vi "RangeDisplay.vi"(7 "Unit":T2, 9 "Range":T1, 11 "error in (no error)":errorcluster) -> (6 "Display":string, 10 "Range":T1, 15 "error out":errorcluster)   [LabVIEW 2014, in "FH 55.lvlib"]
doc: "Dieses VI gibt für die Range (abhängig von der Einheit) denn Zahlenwert für den Display zurück.\n\n\nThis VI gives for the range (depending on the unit) a numerical value for the display back."
uses:
  FH 55.lvlib
  TypeDef/Range.ctl
  TypeDef/Unit.ctl
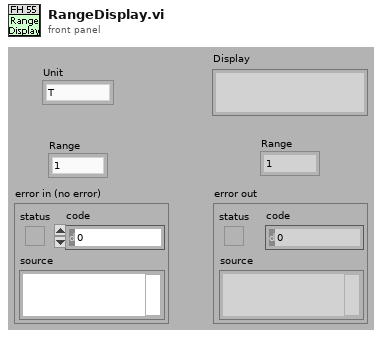
[diagram p1: front panel]
types:
  T1 = typedef "FH 55.lvlib/Range.ctl" = enum16{"1", "2", "3", "4", "5", "6", "7"}
  T2 = typedef "FH 55.lvlib/Unit.ctl" = enum16{"T", "G", "A/m"}
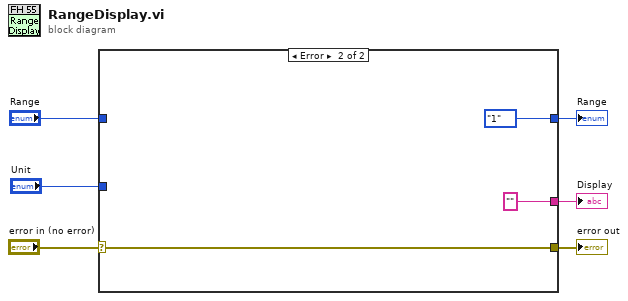
[diagram p0: block diagram]
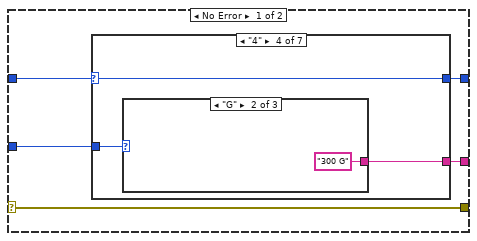
[diagram p2: hidden frame]
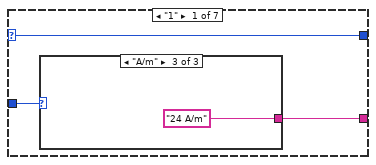
[diagram p3: hidden frame]
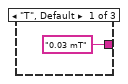
[diagram p4: hidden frame]
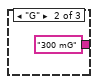
[diagram p5: hidden frame]
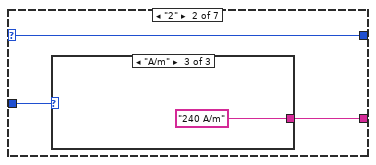
[diagram p6: hidden frame]
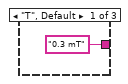
[diagram p7: hidden frame]
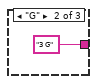
[diagram p8: hidden frame]
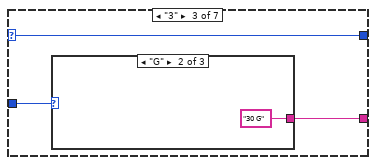
[diagram p9: hidden frame]
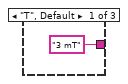
[diagram p10: hidden frame]
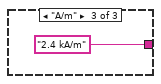
[diagram p11: hidden frame]
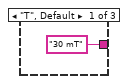
[diagram p12: hidden frame]
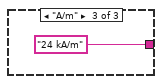
[diagram p13: hidden frame]
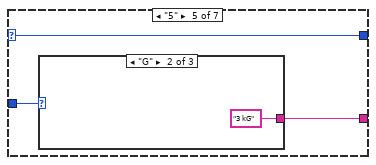
[diagram p14: hidden frame]
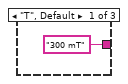
[diagram p15: hidden frame]
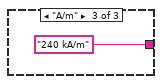
[diagram p16: hidden frame]
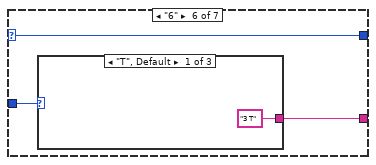
[diagram p17: hidden frame]
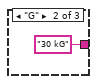
[diagram p18: hidden frame]
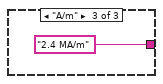
[diagram p19: hidden frame]
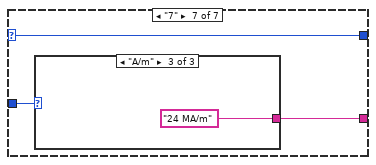
[diagram p20: hidden frame]
diagram:
  n1 = case shown="Error" "error in (no error)" {
    selector: "error in (no error)" -> [w8 w56]
    tunnel: [w8 w56] -> w5
    tunnel: [w11 Range."1" ("Range")] -> w1
    tunnel: "Unit" -> [w7 _]
    tunnel: [w10 ""] -> w3
    tunnel: "Range" -> [w9 _]
    frame No Error {
      n2 = case shown="\"4\"" w9 {
        selector: w9 -> [w14 w20 w26 w32 w38 w44 w50]
        tunnel: [w14 w20 w26 w32 w38 w44 w50] -> w11
        tunnel: [w13 w19 w25 w31 w37 w43 w49] -> w10
        tunnel: w7 -> [w12 w18 w24 w30 w36 w42 w48]
        frame "1" {
          n3 = case shown="\"A/m\"" w12 {
            tunnel: ["0.03 mT" "300 mG" "24 A/m"] -> w13
            frame "T", Default {
            }
            frame "G" {
            }
            frame "A/m" {
            }
          }
        }
        frame "2" {
          n4 = case shown="\"A/m\"" w18 {
            tunnel: ["0.3 mT" "3 G" "240 A/m"] -> w19
            frame "T", Default {
            }
            frame "G" {
            }
            frame "A/m" {
            }
          }
        }
        frame "3" {
          n5 = case shown="\"G\"" w24 {
            tunnel: ["3 mT" "30 G" "2.4 kA/m"] -> w25
            frame "T", Default {
            }
            frame "G" {
            }
            frame "A/m" {
            }
          }
        }
        frame "4" {
          n6 = case shown="\"G\"" w30 {
            tunnel: ["30 mT" "300 G" "24 kA/m"] -> w31
            frame "T", Default {
            }
            frame "G" {
            }
            frame "A/m" {
            }
          }
        }
        frame "5" {
          n7 = case shown="\"G\"" w36 {
            tunnel: ["300 mT" "3 kG" "240 kA/m"] -> w37
            frame "T", Default {
            }
            frame "G" {
            }
            frame "A/m" {
            }
          }
        }
        frame "6" {
          n8 = case shown="\"T\", Default" w42 {
            tunnel: ["3 T" "30 kG" "2.4 MA/m"] -> w43
            frame "T", Default {
            }
            frame "G" {
            }
            frame "A/m" {
            }
          }
        }
        frame "7" {
          n9 = case shown="\"A/m\"" w48 {
            tunnel: ["30 T" "300 kG" "24 MA/m"] -> w49
            frame "T", Default {
            }
            frame "G" {
            }
            frame "A/m" {
            }
          }
        }
      }
    }
    frame Error {
    }
  }
  "error out" <- w5
  "Range" <- w1
  "Display" <- w3
